vi "initializer_load_vali.vi"(6 "LUA Validation File":path, 10 "Parameters Tree":refnum<vi>) -> (2 "Vali File Loaded":bool, 3 "# Lines":i32)   [LabVIEW 2019]
uses:
  lib/libSpecValiReader/libSpecValiReader.lvlib
  lib/libSimulationControl/libSimulationControl.lvlib
panel:
  # "*******************************************************************\nBiogas Plant Control\n\nAuthor: Paul Zügel\nGCSC-Frankfurt am Main 2020\n\n*******************************************************************"
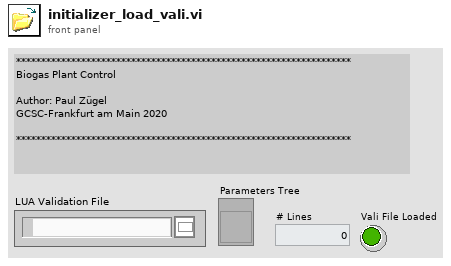
[diagram p1: front panel]
types:
  T1 = cluster{string, string[], "Child Tag":string, i32, "Child Only?":bool, i32}
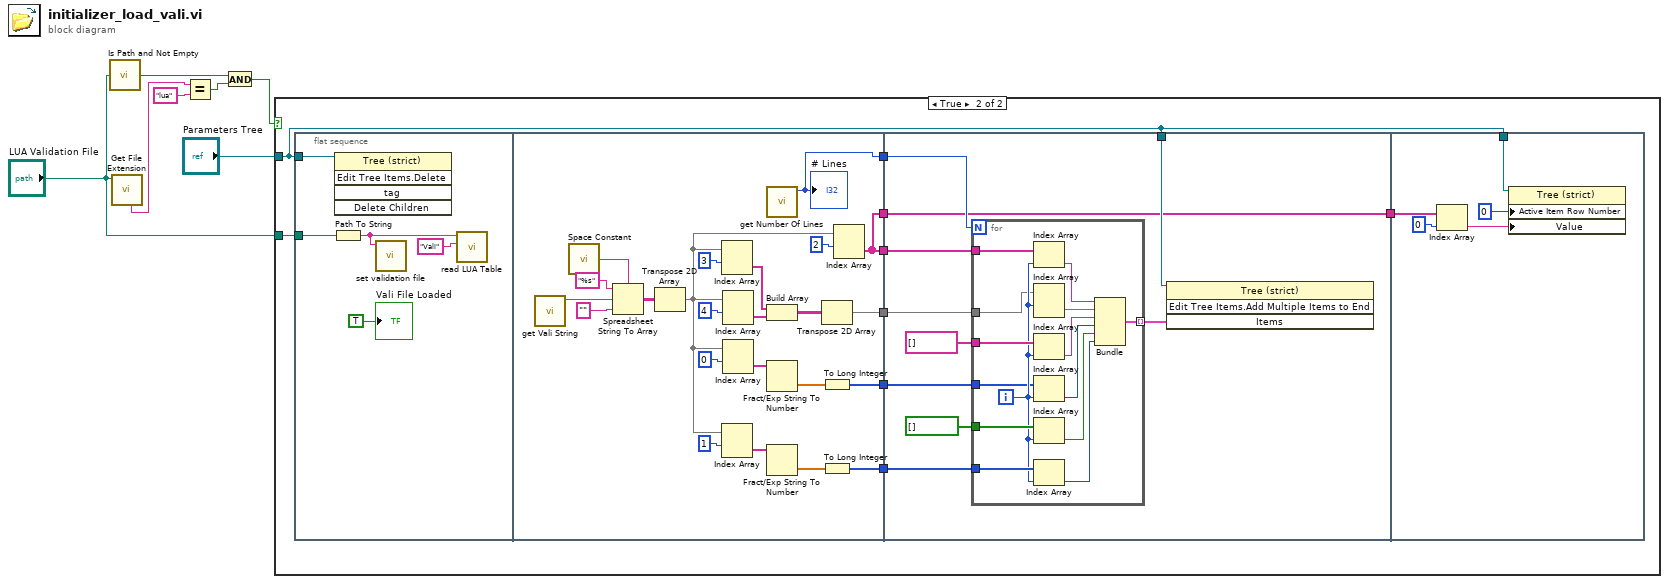
[diagram p0: block diagram]
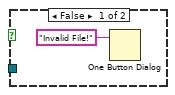
[diagram p2: hidden frame]
diagram:
  n1 = call <vilib>:"Is Path and Not Empty.vi"("path"="LUA Validation File") -> ("Is Path and Not Empty?"=w3:bool)  [unwired: 4 in]
  n2 = call <vilib>:"Get File Extension.vi"("file"="LUA Validation File") -> ("unmodified file extension"=w6:string)  [unwired: 6 in, 4 out]
  n3 = Equal?(x=w6, y="lua") -> (x = y?=w2:bool)
  n4 = And(x=w3, y=w2) -> (x .and. y?=w1:bool)
  n5 = case shown="True" w1 {
    tunnel: "Parameters Tree" -> [_ w10]
    tunnel: "LUA Validation File" -> [_ w9]
    frame False {
      n6 = One Button Dialog(message="Invalid File!") -> ()  [unwired: 1 in, 1 out]
    }
    frame True {
      n7 = flat-sequence {
        tunnel: w10 -> [w21]
        tunnel: w9 -> [w20]
        tunnel: [w23] -> w17
        tunnel: [w38] -> w16
        tunnel: [w34] -> w15
        tunnel: [w27] -> w14
        tunnel: [w27] -> w13
        tunnel: [w25] -> w12
        tunnel: w17 -> [w52]
        tunnel: w10 -> [w51]
        tunnel: w16 -> [w50]
        tunnel: w15 -> [w49]
        tunnel: w14 -> [w48]
        tunnel: [w47] -> w11
        tunnel: w13 -> [w47]
        tunnel: w12 -> [w46]
        tunnel: w10 -> [w72]
        tunnel: w11 -> [w71]
        frame #0 {
          n8 = Path To String(path=w20) -> (string=w18:string)
          n9 = invoke on="Invoke Node" class="Tree (strict)" method="Edit Tree Items.Delete"(reference=w21) -> ()  [unwired: 4 in, 5 out]
          n10 = call "set validation file.vi"("val_file"=w18) -> ()  [unwired: 10 in, 1 out]
          n11 = call "read LUA Table.vi"("vali_or_spec"="Vali" ("spec_filename"), "filename"=w18) -> ()  [unwired: 8 in, 2 out]
          "Vali File Loaded" <- TRUE ("Vali File Loaded")
        }
        frame #1 {
          n12 = call "get Vali String.vi"() -> ("function return"=w24:string)  [unwired: 10 in, 1 out]
          n13 = call <vilib>:"Space Constant.vi"() -> ("String"=w42:string)
          n14 = Spreadsheet String To Array(delimiter (Tab)=w42, format string="%s", spreadsheet string=w24, array type (2D Dbl)="") -> (array=w43:string[][])
          n15 = Transpose 2D Array(2D array=w43) -> (transposed array=w31:string[][])
          n16 = Index Array(array=w31, index (row)=3) -> (element=w29:string[])  [unwired: 1 in]
          n17 = Index Array(array=w31, index (row)=1) -> (element=w36:string[])  [unwired: 1 in]
          n18 = Index Array(array=w31, index (row)=4) -> (element=w28:string[])  [unwired: 1 in]
          n19 = Index Array(array=w31, index (row)=0) -> (element=w40:string[])  [unwired: 1 in]
          n20 = call "get Number Of Lines.vi"() -> ("function return"=w23:i32)  [unwired: 10 in, 1 out]
          "# Lines" <- w23
          n21 = Build Array(w29, w28) -> (w26:string[][])
          n22 = Fract/Exp String To Number(string=w40) -> (number=w39:dbl[])  [unwired: 3 in, 1 out]
          n23 = Fract/Exp String To Number(string=w36) -> (number=w35:dbl[])  [unwired: 3 in, 1 out]
          n24 = Transpose 2D Array(2D array=w26) -> (transposed array=w25:string[][])
          n25 = To Long Integer(number=w39) -> (32bit integer=w38:i32[])
          n26 = To Long Integer(number=w35) -> (32bit integer=w34:i32[])
          n27 = Index Array(array=w31, index (row)=2) -> (element=w27:string[])  [unwired: 1 in]
        }
        frame #2 {
          n28 = for {
            N: w52 -> [_]
            tunnel: w48 -> [w69]
            tunnel: string[] [] ("Child Tag") -> [w68]
            tunnel: w50 -> [w56]
            tunnel: bool[] [] ("Child Only?") -> [w67]
            tunnel: w49 -> [w66]
            tunnel: [w60] -> w55 mode=indexing
            tunnel: w46 -> [w58]
            i -> [w59]
            n29 = Index Array(array=w69, index=w59) -> (element=w65:string)
            n30 = Index Array(array=w58, index (row)=w59) -> (element=w57:string[])  [unwired: 1 in]
            n31 = Index Array(array=w68, index=w59) -> (element=w64:string)
            n32 = Index Array(array=w56, index=w59) -> (element=w63:i32)
            n33 = Index Array(array=w67, index=w59) -> (element=w62:bool)
            n34 = Index Array(array=w66, index=w59) -> (element=w61:i32)
            n35 = Bundle(w65, w57, "Child Tag"=w64, w63, "Child Only?"=w62, w61) -> (w60:T1)  [unwired: 1 in]
          }
          n36 = invoke on="Invoke Node" class="Tree (strict)" method="Edit Tree Items.Add Multiple Items to End"(reference=w51, "Items"=w55) -> ()  [unwired: 2 in, 4 out]
        }
        frame #3 {
          n37 = Index Array(array=w71, index=0) -> (element=w70:string)
          n38 = property on="Property Node" class="Tree (strict)"(reference=w72, "Active Item Row Number"=0 ("Active Item:Row Number"), "Value"=w70) -> ()  [unwired: 1 in, 2 out]
        }
      }
    }
  }
